vi "Periodic Tasks.vi"(8 "error in":errorcluster) -> ()   [LabVIEW 2017]
doc: "This VI runs in parallel to other tasks. It can contain as many user-defined periodic loops as you need. These can carry out PID or other sorts of timed response."
uses:
  <vilib>/Rock Robotics/WPI/Utilities/WPI_GetSetVariantRefNum.vi
panel:
  in  "Disable PID":bool
  out "Chart":cluster{"Setpoint":dbl, "Process variable":dbl}(graph)
  in  "Smoothly Override":bool
  out "output":dbl
  in  "Reset encoder":bool
  in  "Gains":T1={"proportional gain (Kc)"=0.6, "integral time (Ti, min)"=0.005, "derivative time (Td, min)"=0.0} {"derivative time (Td, min)" format="%.8f"; "integral time (Ti, min)" format="%.8f"; "proportional gain (Kc)" format="%.8f"}
  in  "Range":cluster{"output high":dbl, "output low":dbl}={"output high"=0.9, "output low"=0.05} {"output low" format="%.2f"; "output high" format="%.2f"}
  in  "Integral Range":dbl=25.0
  in  "Disable Range":dbl
  in  "Elevator Setpoint":dbl
  out "Distance":dbl(slide) scale=0.0..100.0
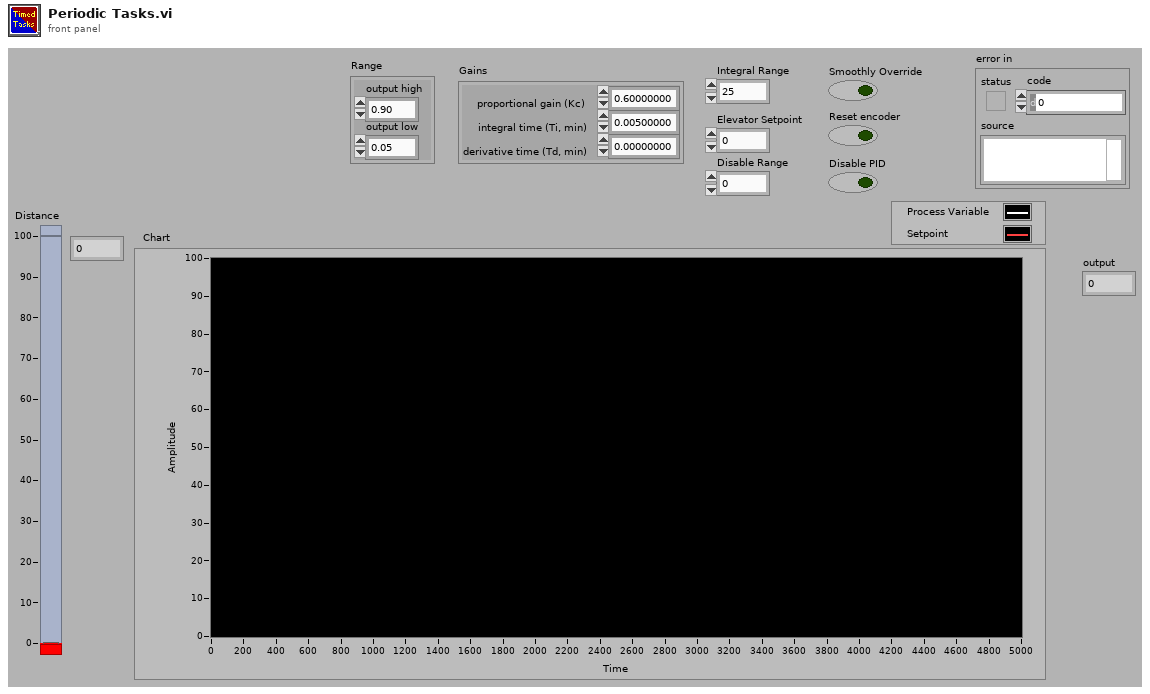
[diagram p1: front panel]
types:
  T1 = cluster{"proportional gain (Kc)":dbl, "integral time (Ti, min)":dbl, "derivative time (Td, min)":dbl}
  T2 = typedef "WPI_JoystickDevRef.ctl" = cluster{"Device":T3}
  T3 = typedef "WPI_JoystickDeviceEnum.ctl" = enum16{"USB 0", "USB 1", "USB 2", "USB 3", "USB 4", "USB 5"}
  T4 = typedef "WPI_MotorControlDeviceRef.ctl" = cluster{"DeviceStatus":errorcluster, "Type":T5, "PWM":cluster{"PWM Channel":T6, "DeadBand":T7}, "CAN":cluster{"Device Number":u8, "SetOutput VI Ref":variant, "GetOutput VI Ref":variant, "Enable VI Ref":variant, "Disable VI Ref":variant, "Data":variant}, "Invert":bool, "DIO PWM":cluster{"PWM \"Enable\" Channel":T6, "DIOChannel":T8, "PWM Rate":dbl}}
  T5 = typedef "WPI_MotorControlType.ctl" = enum16{"PWM", "CAN", "DIO PWM"}
  T6 = typedef "FPGA_DIOPWMChannel.ctl" = enum8{"PWM 0", "PWM 1", "PWM 2", "PWM 3", "PWM 4", "PWM 5", "PWM 6", "PWM 7", "PWM 8", "PWM 9", "PWM MXP 0", "PWM MXP 1", "PWM MXP 2", "PWM MXP 3", "PWM MXP 4", "PWM MXP 5", "PWM MXP 6", "PWM MXP 7", "PWM MXP 8", "PWM MXP 9", "Invalid"}
  T7 = typedef "WPI_PWMDeadband.ctl" = cluster{"Name":string, "maxPositivePwm":i32, "minPositivePwm":i32, "centerPwm":i32, "maxNegativePwm":i32, "minNegativePwm":i32, "angularRange":u16}
  T8 = typedef "FPGA_DIOChannel.ctl" = enum8{"DIO 0", "DIO 1", "DIO 2", "DIO 3", "DIO 4", "DIO 5", "DIO 6", "DIO 7", "DIO 8", "DIO 9", "DIO MXP 0", "DIO MXP 1", "DIO MXP 2", "DIO MXP 3", "DIO MXP 4", "DIO MXP 5", "DIO MXP 6", "DIO MXP 7", "DIO MXP 8", "DIO MXP 9", "DIO MXP 10", "DIO MXP 11", "DIO MXP 12", "DIO MXP 13", "DIO MXP 14", "DIO MXP 15", "SPI Port CS1", "SPI Port CS2", "SPI Port CS3", "SPI Port MISO", "SPI Port MOSI", "Invalid"}
  T9 = typedef "WPI_EncoderDevRef.ctl" = cluster{"DevStatus":errorcluster, "EncoderIndex":T10, "CounterIndex":T11, "DistancePerCount":dbl, "Decoding Type":T12}
  T10 = typedef "FPGA_EncoderIdx.ctl" = enum8{"Enc 0", "Enc 1", "Enc 2", "Enc 3", "Enc 4", "Enc 5", "Enc 6", "Enc 7", "Invalid"}
  T11 = typedef "FPGA_CounterCtrSystemIndex.ctl" = enum8{"Ctr 0", "Ctr 1", "Ctr 2", "Ctr 3", "Ctr 4", "Ctr 5", "Ctr 6", "Ctr 7", "Invalid"}
  T12 = typedef "WPI_EncoderType.ctl" = enum16{"1x", "2x", "4x"}
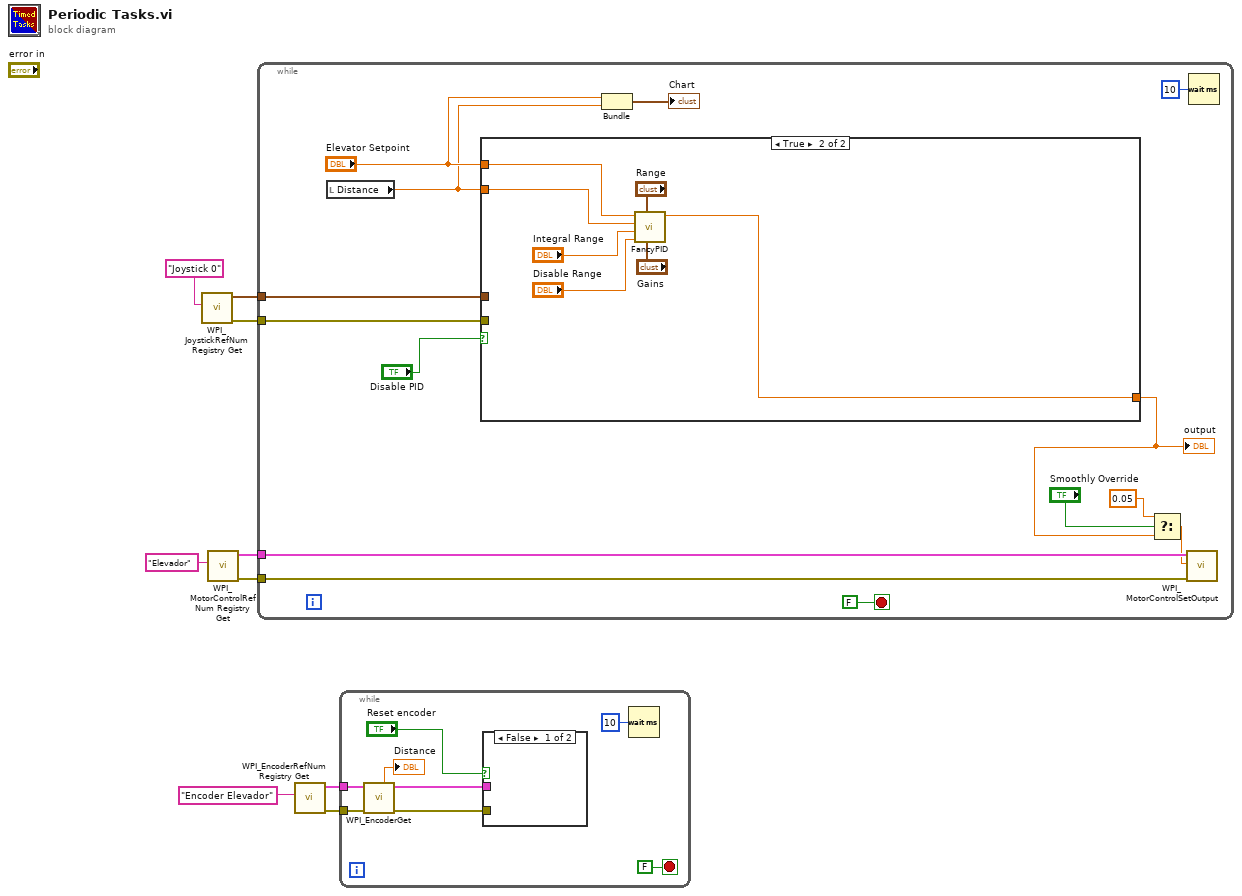
[diagram p0: block diagram]
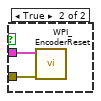
[diagram p2: hidden frame]
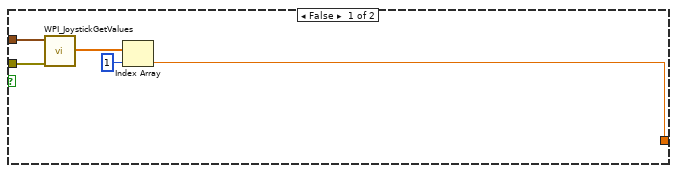
[diagram p3: hidden frame]
diagram:
  n1 = call <vilib>:"WPI_JoystickRefNum Registry Get.vi"("refnum name"="Joystick 0") -> ("error out"=w2:errorcluster, "JoystickDevRef"=w1:T2)  [unwired: 9 in]
  n2 = call <vilib>:"WPI_MotorControlRefNum Registry Get.vi"("refnum name"="Elevador") -> ("error out"=w7:errorcluster, "MotorControlDevRef"=w8:T4)  [unwired: 9 in]
  n3 = while {
    tunnel: w8 -> [w23]
    tunnel: w7 -> [w22]
    tunnel: w2 -> [w19]
    tunnel: w1 -> [w18]
    stop <- FALSE stop-if-true
    n4 = local read "Distance"() -> (w11:dbl)
    n5 = case shown="True" "Disable PID" {
      tunnel: [w24 w29] -> w16
      tunnel: w19 -> [w28 _]
      tunnel: w18 -> [w27 _]
      tunnel: "Elevator Setpoint" -> [_ w31]
      tunnel: w11 -> [_ w30]
      frame False {
        n6 = call <vilib>:"WPI_JoystickGetValues.vi"("error in (no error)"=w28, "JoystickDevRef"=w27) -> ("Axes"=w26:dbl[])  [unwired: 5 in, 4 out]
        n7 = Index Array(array=w26, index=1) -> (element=w24:dbl)
      }
      frame True {
        n8 = call "FancyPID.vi"("Gains"="Gains", "Range"="Range", "Disable Range"="Disable Range", "Integral Range"="Integral Range", "Process variable"=w30, "Setpoint"=w31) -> ("output"=w29:dbl)  [unwired: 5 in]
      }
    }
    "output" <- w16
    n9 = Bundle("Elevator Setpoint"="Elevator Setpoint", "Distance"=w11) -> (→"Chart":cluster{"Elevator Setpoint":dbl, "Distance":dbl})  [unwired: 1 in]
    n10 = Select(t=0.05, s="Smoothly Override", f=w16) -> (s? t:f=w15:dbl)
    n11 = call <vilib>:"WPI_MotorControlSetOutput.vi"("error in (no error)"=w22, "Output"=w15, "MotorControlDevRef"=w23) -> ()  [unwired: 6 in, 3 out]
    n12 = Wait (ms)(milliseconds to wait=u32 10) -> ()  [unwired: 1 out]
  }
  n13 = call <vilib>:"WPI_EncoderRefNum Registry Get.vi"("refnum name"="Encoder Elevador") -> ("error out"=w4:errorcluster, "EncoderDevRef"=w5:T9)  [unwired: 9 in]
  n14 = while {
    tunnel: w5 -> [w41]
    tunnel: w4 -> [w40]
    stop <- FALSE stop-if-true
    n15 = call <vilib>:"WPI_EncoderGet.vi"("error in (no error)"=w40, "EncoderDevRef"=w41) -> ("error out"=w37:errorcluster, "Distance"=→"Distance":dbl, "EncoderDevRef"=w38:T9)  [unwired: 4 in, 3 out]
    n16 = case shown="False" "Reset encoder" {
      tunnel: w38 -> [_ w45]
      tunnel: w37 -> [_ w44]
      frame False {
      }
      frame True {
        n17 = call <vilib>:"WPI_EncoderReset.vi"("error in (no error)"=w44, "EncoderDevRef"=w45) -> ()  [unwired: 8 in, 2 out]
      }
    }
    n18 = Wait (ms)(milliseconds to wait=u32 10) -> ()  [unwired: 1 out]
  }
